vi "set channel configuration.vi"(8 "error in":errorcluster, 9 "Channels to create":T1[](array[typedef]), 10 "class path":path, 11 "Application in":refnum<vi>) -> (0 "error out":errorcluster)   [LabVIEW 2013, in "FixedChannelTBModuleDecideFeatures.lvclass"]
uses:
  FixedChannelTBModuleDecideFeatures.lvclass
  channel configuration.ctl
  <vilib>/NI/Tag Bus Module Framework/channel/channel classification.ctl
  <vilib>/NI/Tag Bus/tag/Data Type.ctl
  <vilib>/NI/Tag Bus Module Framework/channel/TBM channel.lvclass
  <vilib>/NI/Tag Bus/tag/tag descriptor.lvclass
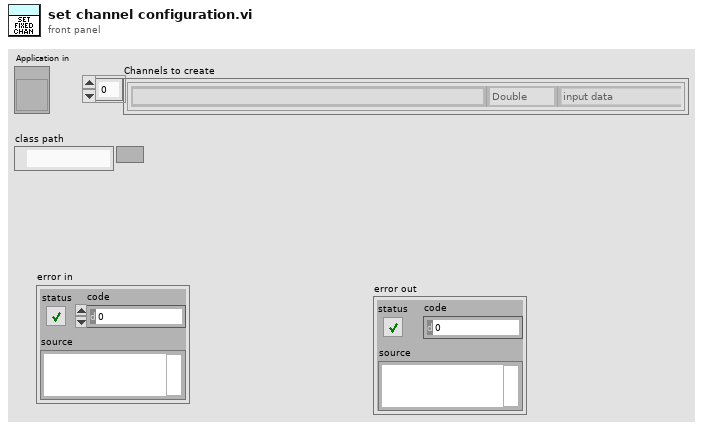
[diagram p1: front panel]
types:
  T1 = typedef "channel configuration.ctl" = cluster{"Name":string, "channel classification":T2, "data type":T3}
  T2 = typedef "TBM channel.lvclass/channel classification.ctl" = enum16{"input data", "output data", "processing parameter", "processing result"}
  T3 = typedef "tag bus.lvlib/tag descriptor.lvclass/Data Type.ctl" = enum16{"Double", "Single", "I64", "I32", "I16", "I8", "U64", "U32", "U16", "U8", "Boolean", "String", "Array of Double", "Array of Single", "Array of I64", "Array of I32", "Array of I16", "Array of I8", "Array of U64", "Array of U32", "Array of U16", "Array of U8", "Array of Boolean", "Array of String"}
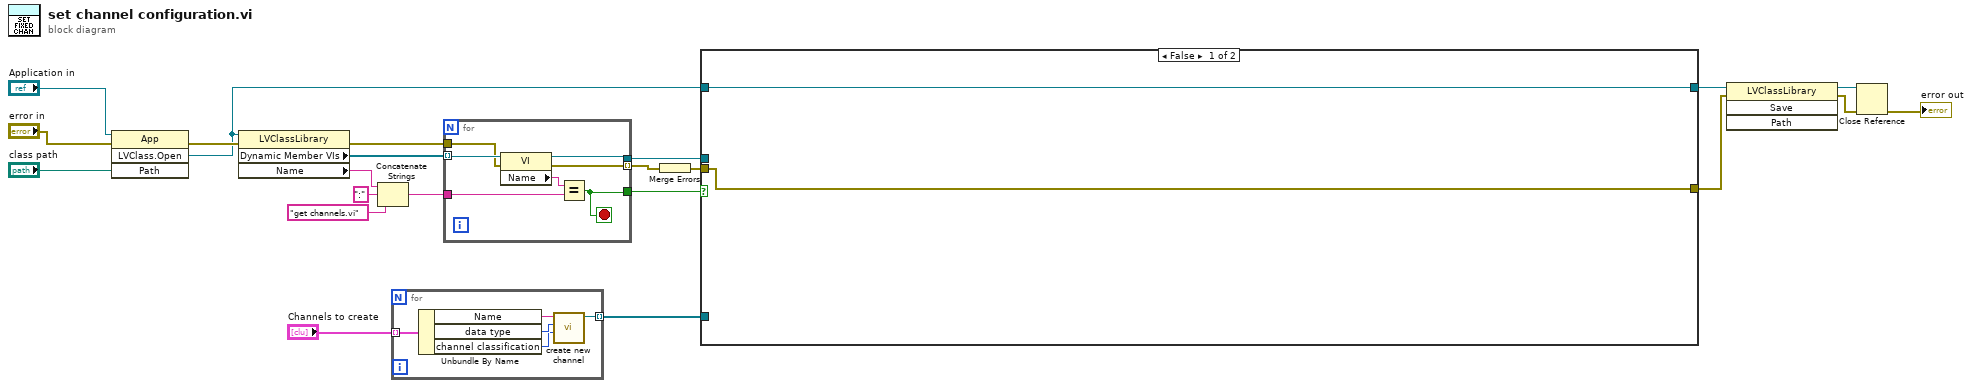
[diagram p0: block diagram]
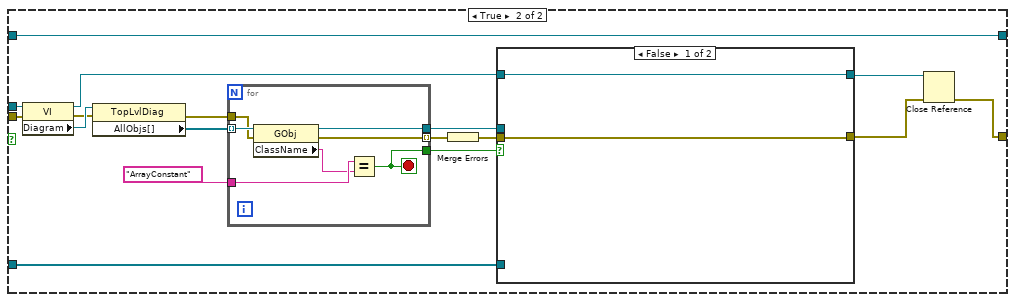
[diagram p2: hidden frame]
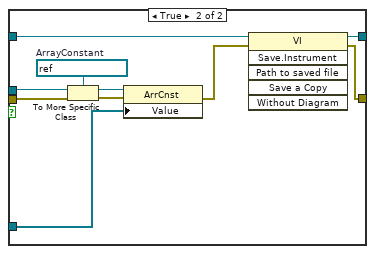
[diagram p3: hidden frame]
diagram:
  n1 = invoke class="App" method="LVClass.Open"(reference="Application in", error in="error in", "Path"="class path") -> (error out=w12:errorcluster, "LVClass.Open"=w6:refnum<vi>)  [unwired: 1 in, 2 out]
  n2 = property class="LVClassLibrary"(reference=w6, error in=w12) -> (error out=w15:errorcluster, "Dynamic Member VIs"=w20:refnum<vi>[], "Name"=w19:string)  [unwired: 1 out]
  n3 = Concatenate Strings(w19, ":" ("string"), "get channels.vi" ("string")) -> (w16:string)
  n4 = for {
    tunnel: "Channels to create" -> [w27] mode=indexing
    tunnel: [w23] -> w8 mode=indexing
    n5 = Unbundle By Name(w27) -> ("Name"=w26:string, "data type"=w25:T3, "channel classification"=w24:T2)
    n6 = call <vilib>:"create new channel.vi"("channel classification"=w24, "data type"=w25, "channel name"=w26) -> ("channel"=w23:refnum<class "TBM channel.lvclass">)  [unwired: 8 in]
  }
  n7 = for {
    tunnel: w20 -> [w34] mode=indexing
    tunnel: w16 -> [w32]
    tunnel: [w31] -> w13
    tunnel: [w30] -> w14
    tunnel: w15 -> [w29]
    tunnel: [w28] -> w11 mode=indexing
    stop <- w31 stop-if-true
    n8 = property class="VI"(reference=w34, error in=w29) -> (reference out=w30:refnum<vi>, error out=w28:errorcluster, "Name"=w33:string)
    n9 = Equal?(x=w33, y=w32) -> (x = y?=w31:bool)
  }
  n10 = Merge Errors(w11) -> (w10:errorcluster)
  n11 = case shown="False" w13 {
    tunnel: w14 -> [_ w53]
    tunnel: w8 -> [_ w47]
    tunnel: w10 -> [w36 w46]
    tunnel: [w36 w37] -> w3
    tunnel: w6 -> [w35 w41]
    tunnel: [w35 w41] -> w5
    frame False {
    }
    frame True {
      n12 = property class="VI"(reference=w53, error in=w46) -> (reference out=w40:refnum<vi>, error out=w45:errorcluster, "Diagram"=w52:refnum<vi>)
      n13 = property class="TopLvlDiag"(reference=w52, error in=w45) -> (error out=w44:errorcluster, "AllObjs[]"=w51:refnum<vi>[])  [unwired: 1 out]
      n14 = for {
        tunnel: w51 -> [w72] mode=indexing
        tunnel: "ArrayConstant" -> [w71]
        tunnel: [w70] -> w48
        tunnel: [w69] -> w49
        tunnel: w44 -> [w67]
        tunnel: [w66] -> w43 mode=indexing
        stop <- w69 stop-if-true
        n15 = property class="GObj"(reference=w72, error in=w67) -> (reference out=w70:refnum<vi>, error out=w66:errorcluster, "ClassName"=w68:string)
        n16 = Equal?(x=w71, y=w68) -> (x = y?=w69:bool)
      }
      n17 = Merge Errors(w43) -> (w42:errorcluster)
      n18 = case shown="False" w49 {
        tunnel: w48 -> [_ w65]
        tunnel: w47 -> [_ w62]
        tunnel: w42 -> [w55 w61]
        tunnel: [w55 w57] -> w38
        tunnel: w40 -> [w54 w59]
        tunnel: [w54 w56] -> w39
        frame False {
        }
        frame True {
          w64 = refnum<vi> refnum  # ArrayConstant
          n19 = To More Specific Class(target class=w64, reference=w65, error in=w61) -> (specific class reference=w63:refnum<vi>, error out=w60:errorcluster)
          n20 = property class="ArrCnst"(reference=w63, error in=w60, "Value"=w62) -> (error out=w58:errorcluster)  [unwired: 1 out]
          n21 = invoke class="VI" method="Save.Instrument"(reference=w59, error in=w58) -> (reference out=w56:refnum<vi>, error out=w57:errorcluster)  [unwired: 4 in, 4 out]
        }
      }
      n22 = Close Reference(reference=w39, error in (no error)=w38) -> (error out=w37:errorcluster)
    }
  }
  n23 = invoke class="LVClassLibrary" method="Save"(reference=w5, error in=w3) -> (reference out=w4:refnum<vi>, error out=w2:errorcluster)  [unwired: 2 in, 2 out]
  n24 = Close Reference(reference=w4, error in (no error)=w2) -> (error out=→"error out":errorcluster)
